vi "Get LabVIEW Class Version.vi"(8 "error in":errorcluster, 11 "File Info in":T1) -> (0 "error out":errorcluster, 3 "File Info out":T1)   [LabVIEW 2020, in "Peer Review.lvclass"]
uses:
  TypeDefs/File Info.ctl
  TypeDefs/File State.ctl
  TypeDefs/VI Type.ctl
  Peer Review.lvclass
  Peer Review.lvclass/Peer Review.ctl
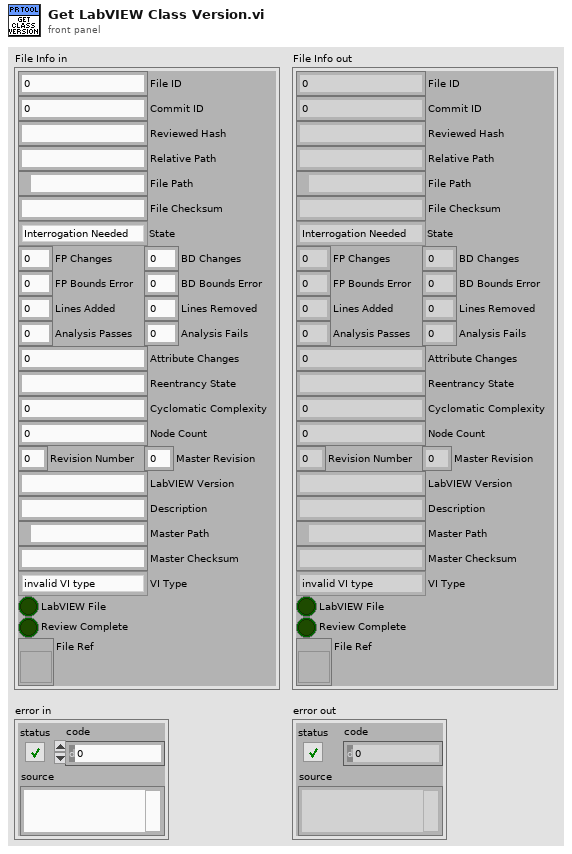
[diagram p1: front panel]
types:
  T1 = typedef "Peer Review.lvclass/File Info.ctl" = cluster{"File ID":i32, "Commit ID":i32, "Reviewed Hash":string, "Relative Path":string, "File Path":path, "File Checksum":string, "State":T2, "FP Changes":i32, "BD Changes":i32, "FP Bounds Error":dbl, "BD Bounds Error":dbl, "Lines Added":i32, "Lines Removed":i32, "Analysis Passes":i32, "Analysis Fails":i32, "Attribute Changes":i32, "Reentrancy State":string, "Cyclomatic Complexity":i32, "Node Count":i32, "Revision Number":u32, "LabVIEW Version":string, "Description":string, "Master Path":path, "Master Checksum":string, "VI Type":T3, "LabVIEW File":bool, "Review Complete":bool, "File Ref":refnum<vi>, "Master Revision":u32}
  T2 = typedef "Peer Review.lvclass/File State.ctl" = enum16{"Interrogation Needed", "Modified", "Deleted", "Added", "Matches Previous", "No Changes", "Moved", "Empty File"}
  T3 = typedef "Peer Review.lvclass/VI Type.ctl" = enum32{"invalid VI type", "Standard VI", "Control VI", "Global VI", "Polymorphic VI", "Configuration VI", "SubSystem", "Facade VI", "Method VI", "Statechart Diagram VI"}
  T4 = enum16{"open", "replace", "create", "open or create", "replace or create", "replace or create with confirmation"}
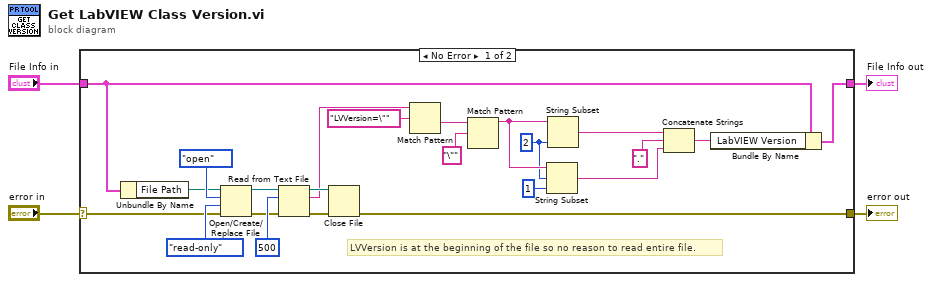
[diagram p0: block diagram]
diagram:
  n1 = case shown="No Error" "error in" {
    selector: "error in" -> [w7 w29]
    tunnel: [w5 w29] -> w4
    tunnel: "File Info in" -> [w27 w28]
    tunnel: [w26 w28] -> w1
    frame No Error {
      w21 = 2 ("length (rest)")
      # "LVVersion is at the beginning of the file so no reason to read entire file."
      n2 = Unbundle By Name(w27) -> ("File Path"=w8:path)
      n3 = Open/Create/Replace File(file path (use dialog)=w8, error in=w7, operation (0:open)=T4."open", access (0:read/write)=enum16{"read/write", "read-only", "write-only"}."read-only") -> (refnum out=w16:refnum<file>, error out=w15:errorcluster)  [unwired: 2 in, 1 out]
      n4 = Read from Text File(file (use dialog)=w16, count=500, error in=w15) -> (refnum out=w14:refnum<file>, text=w11:string, error out=w13:errorcluster)  [unwired: 1 in, 1 out]
      n5 = Close File(refnum=w14, error in=w13) -> (error out=w5:errorcluster)  [unwired: 1 out]
      n6 = Match Pattern(string=w11, regular expression="LVVersion=\"") -> (after substring=w10:string)  [unwired: 1 in, 3 out]
      n7 = Match Pattern(string=w10, regular expression="\"") -> (before substring=w22:string)  [unwired: 1 in, 3 out]
      n8 = String Subset(string=w22, offset (0)=w21, length (rest)=1 ("length (rest)")) -> (substring=w20:string)
      n9 = String Subset(string=w22, length (rest)=w21) -> (substring=w25:string)  [unwired: 1 in]
      n10 = Concatenate Strings(w25, "." ("string"), w20) -> (w6:string)
      n11 = Bundle By Name(cluster=w27, "LabVIEW Version"=w6) -> (w26:T1)
    }
    frame Error {
    }
  }
  "error out" <- w4
  "File Info out" <- w1
